vi "list_items.vi"(8 "error in (no error)":errorcluster, 11 "Table in":refnum<class "InlineTable.lvclass">) -> (0 "error out":errorcluster, 2 "items":string[](array[string]), 3 "Table out":refnum<class "InlineTable.lvclass">)   [LabVIEW 2020, in "toml_edit.lvlib" / "InlineTable.lvclass"]
uses:
  InlineTable.lvclass
  InlineTable.lvclass/InlineTable.ctl
  toml_edit.lvlib
  dragon_toml_32.dll
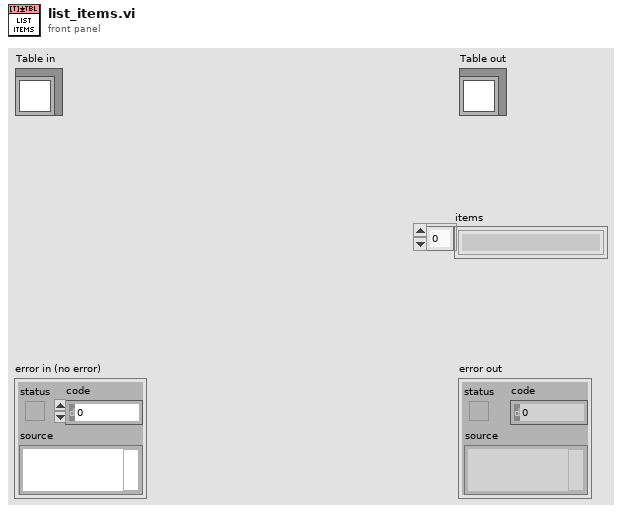
[diagram p1: front panel]
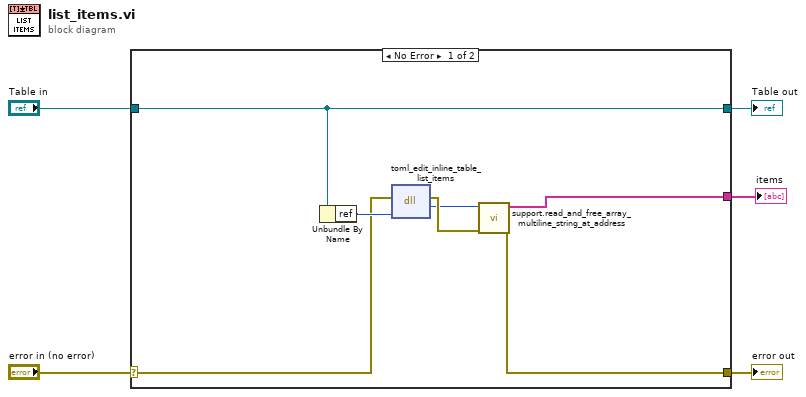
[diagram p0: block diagram]
diagram:
  n1 = case shown="No Error" "error in (no error)" {
    selector: "error in (no error)" -> [w8 w14]
    tunnel: [w7 w14] -> w4
    tunnel: [w9 w13] -> w2
    tunnel: "Table in" -> [w9 w13]
    tunnel: [w6 _] -> w1
    frame No Error {
      n2 = Unbundle By Name(w9) -> ("ref"=w10:u64)
      n3 = dll-call lib="Z:/Share/Projects/jki/toml-edit-labview/lv_src/dragon_toml_*.dll" fn="toml_edit_inline_table_list_items"(error in=w8, "table_ref"=w10) -> (error out=w12:errorcluster, "item_names_ptr"=w11:u64)  [unwired: 3 in, 1 out]
      n4 = call "support.read_and_free_array_multiline_string_at_address.vi"("error in (no error)"=w12, "table_names_ptr"=w11) -> ("error out"=w7:errorcluster, "lines"=w6:string[])  [unwired: 8 in]
    }
    frame Error {
    }
  }
  "error out" <- w4
  "Table out" <- w2
  "items" <- w1
